vi "Write Options.vi"(6 "Options":T1[](array[typedef]), 11 "Car Wash Model in":refnum<class "Car Wash Model.lvclass">) -> (3 "Car Wash Model out":refnum<class "Car Wash Model.lvclass">)   [LabVIEW 2019, in "Car Wash Model.lvclass"]
uses:
  <vilib>/gpm_packages/@cs/Car-wash/Source/Car Wash Model/Car Wash Model/Car Wash Model.lvclass
  <vilib>/gpm_packages/@cs/Car-wash/Source/Application Types/Option Definition.ctl
  <vilib>/gpm_packages/@cs/Car-wash/Source/Car Wash Model/Car Wash Model/Car Wash Model.lvclass/Car Wash Model.ctl
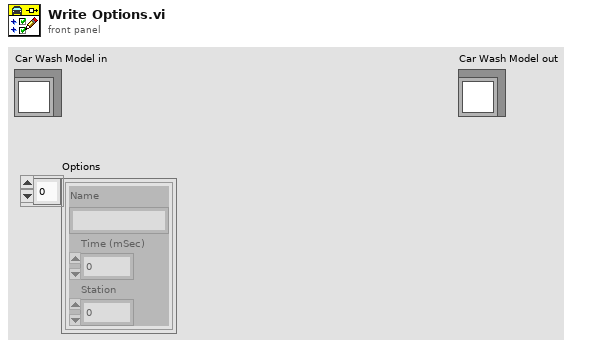
[diagram p1: front panel]
types:
  T1 = typedef "Option Definition.ctl" = cluster{"Name":string, "Time (mSec)":i32, "Station":u8}
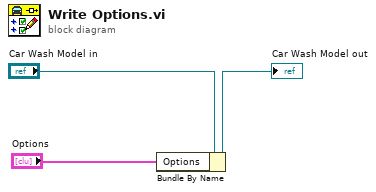
[diagram p0: block diagram]
diagram:
  n1 = Bundle By Name(cluster="Car Wash Model in", "Options"="Options") -> (→"Car Wash Model out":refnum<class "Car Wash Model.lvclass">)
